vi "DBM_Disconnect.vi"(8 "error in (no error)":errorcluster, 11 "DBManager in":refnum<class "DBManager.lvclass">) -> (0 "error out":errorcluster)   [LabVIEW 2015, in "DBManager.lvclass"]
uses:
  DBManager.lvclass
panel:
  # "Connector Pane"
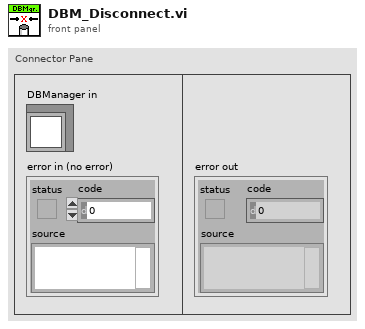
[diagram p1: front panel]
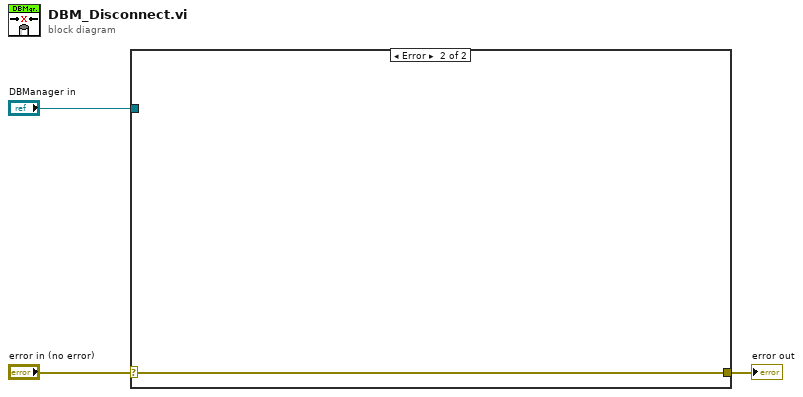
[diagram p0: block diagram]
diagram:
  n1 = case shown="Error" "error in (no error)" {
    selector: "error in (no error)" -> [w4 w5]
    tunnel: [w4 w5] -> w2
    tunnel: "DBManager in" -> [_ _]
    frame No Error {
      # "Wire the error cluster across even in the \"No Error\"\ncase so that warnings get propagated."
    }
    frame Error {
    }
  }
  "error out" <- w2
